vi "1L01-seriegenP.vi"(1 "Pas":dbl, 2 "x_deb":dbl, 3 "Nb":i32) -> (0 "X":dbl[](array[numeric]))   [LabVIEW 2010, in "lv_01.lvlib"]
doc: "Ce VI génère une série (tableau 1D) X à partir des scalaires Nb (nombre de points), Xdeb (valeur de départ), Xfin (Pas)"
uses:
  lv_01.lvlib
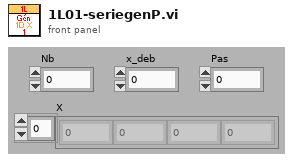
[diagram p1: front panel]
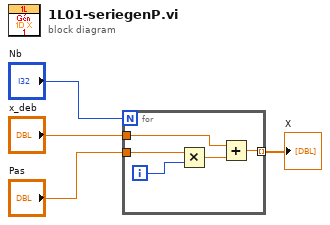
[diagram p0: block diagram]
diagram:
  n1 = for {
    N: "Nb" -> [_]
    tunnel: [w7] -> w4 mode=indexing
    tunnel: "x_deb" -> [w6]
    tunnel: "Pas" -> [w5]
    i -> [w8]
    n2 = Multiply(x=w5, y=w8) -> (x*y=w9:dbl)
    n3 = Add(x=w6, y=w9) -> (x+y=w7:dbl)
  }
  "X" <- w4
